vi "Run Javascript.vi"(0 "Display State In":T1={"WebView2 Ref"=refnum, "event callback refnum"=refnum, "Events"={"Navigation Complete Event"=refnum, "Source Changed Event"=refnum, "Document Title Changed Event"=refnum, "Status Bar Text Changed"=refnum, "Web Message Received"=refnum, "Window Close Requested"=refnum, "DOM Loaded"=refnum, "Navigation Started Event"=refnum}, "Paths"={"Webview2 Native"=path "C:/Users/kleins/Desktop/webview2/microsoft.web.webview2.1.0.1370.28/build/native", "Edge Application"=path "", "User Data"=path ""}, "Environment Options"={"additionalBrowserArguments"="", "language"="", "targetCompatibleBrowserVersion"="", "allowSingleSignOnUsingOSPrimaryAccount"=FALSE}}, 5 "javaScript":string, 7 "Decode Result":bool=TRUE, 9 "Container State":T5, 11 "error in (no error)":errorcluster) -> (4 "Display State Out":T1={"WebView2 Ref"=refnum, "event callback refnum"=refnum, "Events"={"Navigation Complete Event"=refnum, "Source Changed Event"=refnum, "Document Title Changed Event"=refnum, "Status Bar Text Changed"=refnum, "Web Message Received"=refnum, "Window Close Requested"=refnum, "DOM Loaded"=refnum, "Navigation Started Event"=refnum}, "Paths"={"Webview2 Native"=path "C:/Users/kleins/Desktop/webview2/microsoft.web.webview2.1.0.1370.28/build/native", "Edge Application"=path "", "User Data"=path ""}, "Environment Options"={"additionalBrowserArguments"="", "language"="", "targetCompatibleBrowserVersion"="", "allowSingleSignOnUsingOSPrimaryAccount"=FALSE}}, 6 "Result":string, 15 "error out":errorcluster)   [LabVIEW 2020, in "WebView2 Control.xctl"]
uses:
  WebView2 Control.xctl
  <vilib>/_xctls/Container State.ctl
  State.ctl
  E:/Labview/LV 2020/Libs/WebView2/LV-WebView2/Source/Libs/Microsoft.Web.WebView2.WinForms.dll
  Libs/Microsoft.Web.WebView2.WinForms.dll
  Events.ctl
  Navigation Event Data.ctl
  Source Changed Event Data.ctl
  Navigation Start Event Data.ctl
  E:/Labview/LV 2020/Libs/WebView2/LV-WebView2/Source/Libs/Microsoft.Web.WebView2.Core.dll
  Libs/Microsoft.Web.WebView2.Core.dll
  Paths.ctl
  Core Env Options.ctl
  <vilib>/_xctls/XControlSupport.lvlib
panel:
  # "Add Controls & Indicators that form the parameters of the method here. Hook them to the connector pane. Do not delete the controls & indicators that are already hooked to the connector pane.\n \nTo setup the parameters  for this method, right click on this item in the Project Tree & select \"Configure Method...\"."
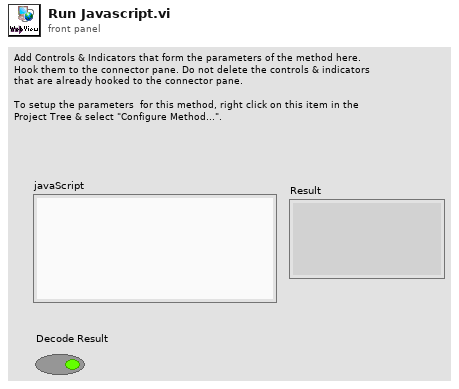
[diagram p1: front panel]
types:
  T1 = typedef "WebView2 Control.xctl/State.ctl" = cluster{"WebView2 Ref":refnum<data-value>, "event callback refnum":refnum<k27>, "Events":T2, "Paths":T3, "Environment Options":T4}
  T2 = typedef "WebView2 Control.xctl/Events.ctl" = cluster{"Navigation Complete Event":refnum<user-event>, "Source Changed Event":refnum<user-event>, "Document Title Changed Event":refnum<user-event>, "Status Bar Text Changed":refnum<user-event>, "Web Message Received":refnum<user-event>, "Window Close Requested":refnum<user-event>, "DOM Loaded":refnum<user-event>, "Navigation Started Event":refnum<user-event>}
  T3 = typedef "WebView2 Control.xctl/Paths.ctl" = cluster{"Webview2 Native":path, "Edge Application":path, "User Data":path}
  T4 = typedef "WebView2 Control.xctl/Core Env Options.ctl" = cluster{"additionalBrowserArguments":string, "language":string, "targetCompatibleBrowserVersion":string, "allowSingleSignOnUsingOSPrimaryAccount":bool}
  T5 = typedef "XControlSupport.lvlib/Container State.ctl" = cluster{"Indicator?":bool, "Run Mode?":bool, " Refnum":refnum<vi>}
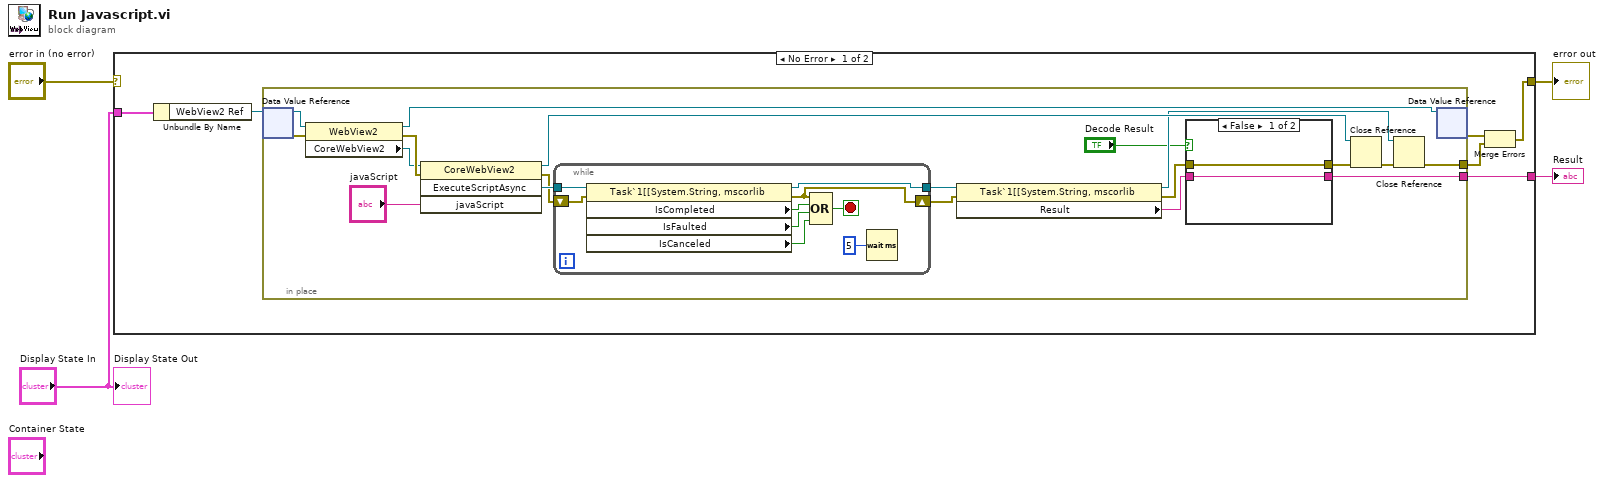
[diagram p0: block diagram]
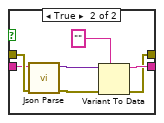
[diagram p2: hidden frame]
diagram:
  n1 = case shown="No Error" "error in (no error)" {
    selector: "error in (no error)" -> [_ w48]
    tunnel: [w9 w48] -> w3
    tunnel: "Display State In" -> [w7 _]
    tunnel: [w5 _] -> w1
    frame No Error {
      n2 = Unbundle By Name(w7) -> ("WebView2 Ref"=w6:refnum<data-value>)
      n3 = in-place {
        in-place-border: [w19] -> w10
        in-place-border: [w17] -> w5
        n4 = in-place-dvr #1(w6) -> (w28:refnum<k24>, w27:errorcluster)
        n5 = property class="WebView2"(reference=w28, error in=w27) -> (reference out=w26:refnum<k24>, error out=w29:errorcluster, "CoreWebView2"=w23:refnum<k24>)
        n6 = invoke class="CoreWebView2" method="ExecuteScriptAsync"(reference=w23, error in=w29, "javaScript"="javaScript") -> (reference out=w24:refnum<k24>, error out=w21:errorcluster, "ExecuteScriptAsync"=w22:refnum<k24>)  [unwired: 1 in, 1 out]
        n7 = while {
          tunnel: w22 -> [w47]
          shift-right: [w45] -> w20
          shift-left: w21 -> [w46]
          tunnel: [w41] -> w16
          stop <- w44 stop-if-true
          n8 = property class="Task`1[[System.String, mscorlib"(reference=w47, error in=w46) -> (reference out=w41:refnum<k24>, error out=w45:errorcluster, "IsCompleted"=w43:bool, "IsFaulted"=w40:bool, "IsCanceled"=w39:bool)
          n9 = Compound Arithmetic op=OR(w45, w43, w40, w39) -> (w44:bool)
          n10 = Wait (ms)(milliseconds to wait=u32 5) -> ()  [unwired: 1 out]
        }
        n11 = property class="Task`1[[System.String, mscorlib"(reference=w16, error in=w20) -> (reference out=w18:refnum<k24>, error out=w13:errorcluster, "Result"=w12:string)
        n12 = case shown="False" "Decode Result" {
          tunnel: [w31 w37] -> w17
          tunnel: [w30 w36] -> w15
          tunnel: w13 -> [w30 w35]
          tunnel: w12 -> [w31 w34]
          frame False {
          }
          frame True {
            n13 = call "Json Parse.vi"("error in (no error)"=w35, "JSON"=w34) -> ("error out"=w33:errorcluster, "variant"=w32:variant)  [unwired: 8 in]
            n14 = Variant To Data(error in=w33, type="", Variant=w32) -> (data=w37:string, error out=w36:errorcluster)
          }
        }
        n15 = Close Reference(reference=w24, error in (no error)=w15) -> (error out=w25:errorcluster)
        n16 = Close Reference(reference=w18, error in (no error)=w25) -> (error out=w19:errorcluster)
        n17 = in-place-dvr #1(w26) -> (w8:errorcluster)  [unwired: 1 out]
      }
      n18 = Merge Errors(w8, w10) -> (w9:errorcluster)
    }
    frame Error {
    }
  }
  "error out" <- w3
  "Result" <- w1
  "Display State Out" <- "Display State In"
